vi "Waveform Data Logger RT Driver VI.vi"(7 "Operation":T1, 11 "Device Reference in":T2 format="%.0x") -> (0 "Error Code":i32)   [LabVIEW 2015, in "Waveform Data Logger Engine.lvlib"]
uses:
  Waveform Data Logger Engine.lvlib
  <vilib>/NI Veristand/Custom Device API/Custom Device Item Ref.ctl
  <vilib>/NI Veristand/Custom Device API/Hardware Interface Driver VI Operation.ctl
  Types/RT Data.ctl
  Types/Inline Waveform Info.ctl
  <vilib>/NI Veristand/Custom Device API/Waveform Data Reference.ctl
  Classes/Waveforms/Waveform Receive/Associated Log.ctl
  <vilib>/NI Veristand/Custom Device API/Custom Device Waveform DataType.ctl
  Types/Channels.ctl
  <vilib>/NI Veristand/Custom Device API/Block Data Reference.ctl
  <vilib>/NI Veristand/Custom Device API/Data Reference.ctl
  Types/System Time.ctl
  Types/Inline Waveform Log Info.ctl
  Shared/Classes/Log File Specifications/Waveform TDMS Log File Specification/Waveform TDMS Log File Specification.lvclass
  Types/Inline Log Waveform.ctl
  Types/Trigger Settings.ctl
  Classes/Triggers/Trigger/Trigger.lvclass
  Types/Log Status.ctl
  Types/Channel.ctl
  Types/Communication.ctl
  Types/Async Status.ctl
  Types/Async State.ctl
  <vilib>/NI Veristand/Custom Device Waveform API/Communication Properties.ctl
  Types/Trigger Event Data.ctl
  Types/Trigger Received.ctl
  Types/New File Event Data.ctl
  Types/Log Queues.ctl
  <vilib>/NI Veristand/Custom Device Tools/Custom Device Utility Library/NI VeriStand - Print Debug String.vi
  <vilib>/Utility/error.llb/Simple Error Handler.vi
  <vilib>/NI VeriStand/Custom Device API/Custom Device API.lvlib
  Classes/Waveforms/Waveform Receive/Waveform Receive.lvclass
  <vilib>/NI Veristand/Custom Device Waveform API/NI_VS Custom Device Waveform API.lvlib
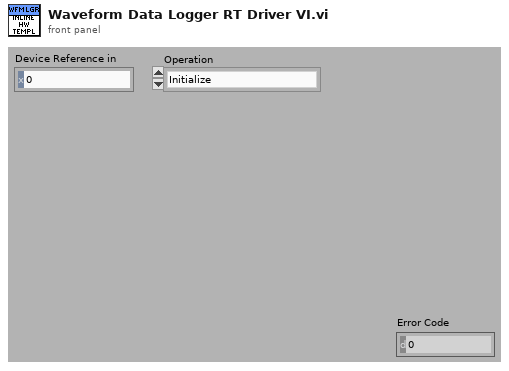
[diagram p1: front panel]
types:
  T1 = typedef "Custom Device API.lvlib/Hardware Interface Driver VI Operation.ctl" = enum16{"Initialize", "Start", "Read Data from HW", "Write Data to HW", "Close"}
  T2 = typedef "Custom Device API.lvlib/Custom Device Item Ref.ctl" = u64
  T3 = typedef "Waveform Data Logger Engine.lvlib/RT Data.ctl" = cluster{"Device Ref":T2, "Waveforms":T4[], "Channels":T8, "Waveform Logs":T12[], "Communication":T16, "error":errorcluster}
  T4 = typedef "Waveform Data Logger Engine.lvlib/Inline Waveform Info.ctl" = cluster{"Waveform Ref in":T2, "Data Ref":T5, "System Name":string, "System Path":string, "Description":string, "Associated Logs":T6[], "Max Pretrigger Time":dbl, "Buffer data?":bool, "Data Type":T7, "GUID":string, "Units":string}
  T5 = typedef "Custom Device API.lvlib/Waveform Data Reference.ctl" = i32
  T6 = typedef "Waveform Data Logger Engine.lvlib/Waveform Receive.lvclass/Associated Log.ctl" = cluster{"Log Index":i32, "Wfm Index":i32}
  T7 = typedef "Custom Device API.lvlib/Custom Device Waveform DataType.ctl" = enum16{"Double", "Complex Double"}
  T8 = typedef "Waveform Data Logger Engine.lvlib/Channels.ctl" = cluster{"Command Chan Refs":T2[], "Command Data Refs":T9[], "Command Values":dbl[], "Status Chan Refs":T2[], "Status Data Refs":T9[], "Status Values":dbl[], "System Time":T11, "Trigger Chan Refs":T2[], "Trigger Data Refs":T9[], "Trigger Values":dbl[]}
  T9 = typedef "Custom Device API.lvlib/Block Data Reference.ctl" = cluster{"Data Reference":T10, "Offset":u64, "Length":u64}
  T10 = typedef "Custom Device API.lvlib/Data Reference.ctl" = i32
  T11 = typedef "Waveform Data Logger Engine.lvlib/System Time.ctl" = cluster{"System Time":timestamp, "Data Reference":T10, "Absolute Time Channel Data Ref":T10, "Get Date-Time Channel Data Ref":T10}
  T12 = typedef "Waveform Data Logger Engine.lvlib/Inline Waveform Log Info.ctl" = cluster{"Node ID":T2, "Log Index":i32, "Log File Spec":refnum<class "Waveform TDMS Log File Specification.lvclass">, "Waveforms":T13[], "Retriggerable":bool, "Allow multiple instances?":bool, "Dependent Logs":i32[], "Ignore Wfm Timestamps?":bool, "File size (bytes)":i64, "Start Trigger":T14, "Stop Trigger":T14, "Timeout":dbl, "Logging Enabled Q":refnum<queue>, "Log Status Q":refnum<queue>, "Logging Enabled":T15, "Start New File":T15, "File Status":T15, "Missed Samples":T15, "TDMS Error Code":T15, "Active Instances":i32}
  T13 = typedef "Waveform Data Logger Engine.lvlib/Inline Log Waveform.ctl" = cluster{"Index":i32, "Name":string, "Decimation":u32}
  T14 = typedef "Waveform Data Logger Engine.lvlib/Trigger Settings.ctl" = cluster{"Node ID":T2, "Node Data Ref":i32, "Path":string, "Trigger":refnum<class "Trigger.lvclass">, "Time":dbl, "Index":i32, "Value":dbl}
  T15 = typedef "Waveform Data Logger Engine.lvlib/Channel.ctl" = cluster{"Index":i32, "Data Ref":T10, "Value":dbl, "Previous Value":dbl}
  T16 = typedef "Waveform Data Logger Engine.lvlib/Communication.ctl" = cluster{"Async Status":refnum<queue>, "Wfm Comm Properties":T17, "Shutdown Event":refnum<user-event>, "Trigger Event":refnum<user-event>, "New File Event":refnum<user-event>, "Log Queues":T18[], "Async VI Ref":refnum<vi>}
  T17 = typedef "NI_VS Custom Device Waveform API.lvlib/Communication Properties.ctl" = cluster{"WPL":cluster{"Custom Queue Size":i32, "Use Custom Queue Size?":bool}}
  T18 = typedef "Waveform Data Logger Engine.lvlib/Log Queues.ctl" = cluster{"Logging Enabled Q":refnum<queue>, "Log Status Q":refnum<queue>}
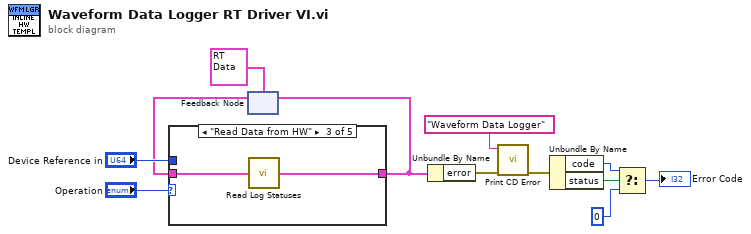
[diagram p0: block diagram]
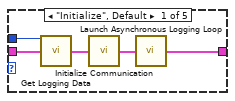
[diagram p2: hidden frame]
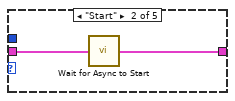
[diagram p3: hidden frame]
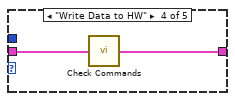
[diagram p4: hidden frame]
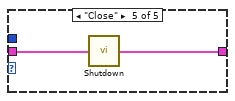
[diagram p5: hidden frame]
diagram:
  n1 = feedback #1(T3 {"Device Ref"=0, "Waveforms"=[], "Channels"={"Command Chan Refs"=[], "Command Data Refs"=[], "Command Values"=[], "Status Chan Refs"=[], "Status Data Refs"=[], "Status Values"=[], "System Time"={"System Time"=timestamp(0 s since 1904-01-01), "Data Reference"=0, "Absolute Time Channel Data Ref"=0, "Get Date-Time Channel Data Ref"=0}, "Trigger Chan Refs"=[], "Trigger Data Refs"=[], "Trigger Values"=[]}, "Waveform Logs"=[], "Communication"={"Async Status"=refnum, "Wfm Comm Properties"={"WPL"={"Custom Queue Size"=0, "Use Custom Queue Size?"=FALSE}}, "Shutdown Event"=refnum, "Trigger Event"=refnum, "New File Event"=refnum, "Log Queues"=[], "Async VI Ref"=refnum}, "error"={"status"=FALSE, "code"=0, "source"=""}} ("RT Data")) -> (w5:T3)
  n2 = case shown="\"Read Data from HW\"" "Operation" {
    tunnel: "Device Reference in" -> [w14 _ _ _ _]
    tunnel: w5 -> [w15 w19 w21 w23 w25]
    tunnel: [w13 w18 w20 w22 w24] -> w10
    frame "Initialize", Default {
      n3 = call "Get Logging Data.vi"("Device Ref in"=w14, "RT Data in"=w15) -> ("RT Data out"=w17:T3)  [unwired: 13 in]
      n4 = call "Initialize Communication.vi"("RT Data in"=w17) -> ("RT Data out"=w16:T3)
      n5 = call "Launch Asynchronous Logging Loop.vi"("RT Data in"=w16) -> ("RT Data out"=w13:T3)
    }
    frame "Start" {
      n6 = call "Wait for Async to Start.vi"("RT Data in"=w19) -> ("RT Data out"=w18:T3)
    }
    frame "Read Data from HW" {
      n7 = call "Read Log Statuses.vi"("RT Data in"=w21) -> ("RT Data out"=w20:T3)
    }
    frame "Write Data to HW" {
      n8 = call "Check Commands.vi"("RT Data"=w23) -> ("RT Data out"=w22:T3)
    }
    frame "Close" {
      n9 = call "Shutdown.vi"("RT Data in"=w25) -> ("RT Data out"=w24:T3)
    }
  }
  n10 = feedback-in #1(w10) -> ()
  n11 = Unbundle By Name(w10) -> ("error"=w4:errorcluster)
  n12 = call "Print CD Error.vi"("error in"=w4, "Your code's public name"="Waveform Data Logger") -> ("error out"=w3:errorcluster)  [unwired: 8 in]
  n13 = Unbundle By Name(w3) -> ("code"=w7:i32, "status"=w9:bool)
  n14 = Select(t=w7, s=w9, f=0) -> (s? t:f=→"Error Code":i32)
